vi "Query Clock Status.vi"(6 "timeout (ms)":i32=5000, 8 "error in":errorcluster, 11 "gRPC ID in":T4) -> (0 "error out":errorcluster, 2 "clocks_status":T1[](array[typedef]), 3 "gRPC ID out":T4)   [LabVIEW 2021, in "CIFManagerClientWrapper.lvlib"]
uses:
  CIFManagerClientWrapper.lvlib
  <vilib>/gRPC/LabVIEW gRPC Library/Shared/grpcId.ctl
  CIF_Manager_client/RPC Messages/cif_manager_ClockStatus.ctl
  CIF_Manager_client/RPC Messages/cif_manager_ClockConversion.ctl
  CIF_Manager_client/RPC Messages/cif_manager_TimePair.ctl
  CIF_Manager_client/CIF_Manager_client.lvlib
  <vilib>/gRPC/LabVIEW gRPC Library/grpc-lvsupport-release.lvlib
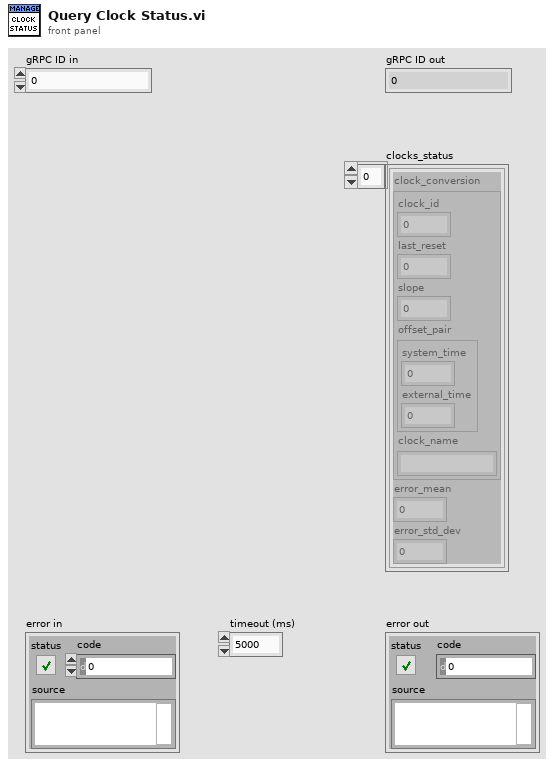
[diagram p1: front panel]
types:
  T1 = typedef "CIF_Manager_client.lvlib/cif_manager_ClockStatus.ctl" = cluster{"clock_conversion":T2, "error_mean":i64, "error_std_dev":i64}
  T2 = typedef "CIF_Manager_client.lvlib/cif_manager_ClockConversion.ctl" = cluster{"clock_id":u32, "last_reset":i64, "slope":dbl, "offset_pair":T3, "clock_name":string}
  T3 = typedef "CIF_Manager_client.lvlib/cif_manager_TimePair.ctl" = cluster{"system_time":i64, "external_time":i64}
  T4 = typedef "grpc-lvsupport-release.lvlib/grpcId.ctl" = u64
  T5 = typedef "CIF_Manager_client.lvlib/cif_manager_QueryClockStatusResponse.ctl" = cluster{"clock_status_array":T6}
  T6 = typedef "CIF_Manager_client.lvlib/cif_manager_ClockStatusArray.ctl" = cluster{"clocks_status":T1[]}
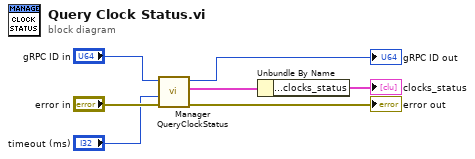
[diagram p0: block diagram]
diagram:
  n1 = call "Manager QueryClockStatus.vi"("error in"="error in", "timeout (ms)"="timeout (ms)", "gRPC ID"="gRPC ID in") -> ("error out"=→"error out":errorcluster, "Response Data"=w2:T5, "gRPC ID out"=→"gRPC ID out":T4)  [unwired: 6 in]
  n2 = Unbundle By Name(w2) -> ("clock_status_array.clocks_status"=→"clocks_status":T1[])
